vi "_luncher.vi"   [LabVIEW 2020]
uses:
  Controller/Controller/Controller.lvclass
  C:/Program Files/National Instruments/LabVIEW 2020/vi.lib/ActorFramework/Actor/Actor.lvclass
  <vilib>/ActorFramework/Actor/Actor.lvclass
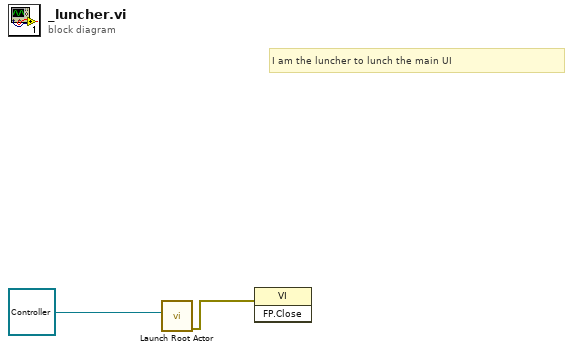
[diagram p0: block diagram]
diagram:
  # "I am the luncher to lunch the main UI"
  n1 = call <vilib>:"Launch Root Actor.vi"("Actor"=refnum<class "Controller.lvclass"> refnum ("Controller.lvlib:Controller.lvclass")) -> ("error out"=w1:errorcluster)  [unwired: 9 in, 1 out]
  n2 = invoke class="VI" method="FP.Close"(error in=w1) -> ()  [unwired: 2 in, 3 out]
